vi "ck_clnt.vi"   [LabVIEW 2012]
uses:
  <vilib>/addons/internet/NI_InternetTK_Common_VIs.lvlib
  <vilib>/addons/internet/NI_InternetTK_Core_VIs.lvlib
types:
  T1 = typedef "CGI Connection Info.ctl" = cluster{"name":string, "type":T2, "session":T3}
  T2 = typedef "CGI Request Type.ctl" = enum16{"cgi", ".spool first", ".spool", ".spool last"}
  T3 = typedef "HTTP Session.ctl" = refnum<k1>
  T4 = typedef "NI_FTP.lvlib/Keyed Array.ctl" = cluster{"keys":string[], "values":string[]}
  T5 = typedef "Cookie.ctl" = cluster{"cookie id":string, "address":string}
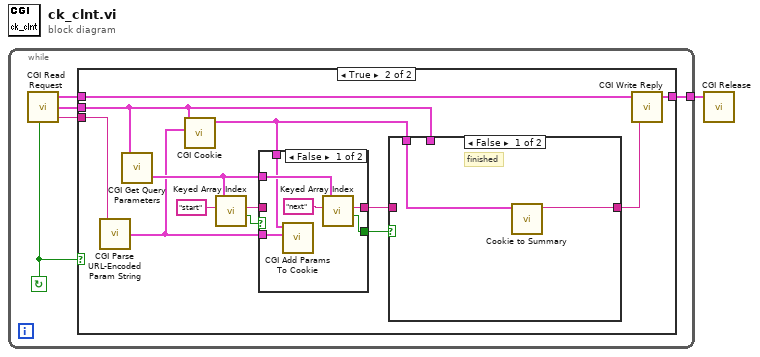
[diagram p0: block diagram]
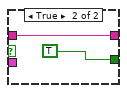
[diagram p3: hidden frame]
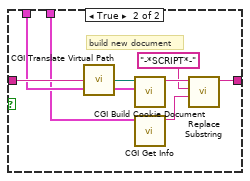
[diagram p4: hidden frame]
diagram:
  n1 = while {
    tunnel: [w2] -> w1
    stop <- w3 continue-if-true
    n2 = call <vilib>:"CGI Read Request.vi"() -> ("valid request?"=w3:bool, "cgi connection info"=w4:T1, "env"=w5:T4, "content"=w6:string)  [unwired: 4 in]
    n3 = case shown="True" w3 {
      tunnel: w4 -> [w7 w14]
      tunnel: [w7 w13] -> w2
      tunnel: w5 -> [_ w9]
      tunnel: w6 -> [_ w12]
      frame False {
      }
      frame True {
        n4 = call <vilib>:"CGI Parse URL-Encoded Param String.vi"("url-encoded param string"=w12) -> ("params"=w10:T4)
        n5 = call <vilib>:"CGI Get Query Parameters.vi"("env"=w9) -> ("query params"=w11:T4)  [unwired: 2 out]
        n6 = call <vilib>:"CGI Cookie.vi"("params"=w10, "env"=w9) -> ("cookie"=w8:T5)  [unwired: 6 in, 3 out]
        n7 = call <vilib>:"Keyed Array Index.vi"("key"="start", "array in"=w11) -> ("valid key"=w17:bool, "value"=w18:string)  [unwired: 3 in, 1 out]
        n8 = case shown="False" w17 {
          tunnel: w18 -> [_ w28]
          tunnel: w11 -> [w25 _]
          tunnel: [w24 TRUE ("valid key")] -> w19
          tunnel: [w23 w28] -> w20
          tunnel: w10 -> [w21 _]
          tunnel: w8 -> [w22 _]
          frame False {
            n9 = call <vilib>:"CGI Add Params To Cookie.vi"("params"=w21, "cookie"=w22) -> ()  [unwired: 8 in, 2 out]
            n10 = call <vilib>:"Keyed Array Index.vi"("key"="next", "array in"=w25) -> ("valid key"=w24:bool, "value"=w23:string)  [unwired: 3 in, 1 out]
          }
          frame True {
          }
        }
        n11 = case shown="False" w19 {
          tunnel: w20 -> [_ w38]
          tunnel: [w30 w35] -> w15
          tunnel: w9 -> [_ w32]
          tunnel: w8 -> [w29 w33]
          frame False {
            # "finished"
            n12 = call "Cookie to Summary.vi"("cookie"=w29) -> ("html summary"=w30:string)  [unwired: 9 in, 1 out]
          }
          frame True {
            # "build new document"
            n13 = call <vilib>:"CGI Translate Virtual Path.vi"("virtual path"=w38) -> ("absolute path"=w37:path)  [unwired: 1 in]
            n14 = call <vilib>:"CGI Build Cookie Document.vi"("cookie"=w33, "document path"=w37) -> ("parsed document"=w36:string)  [unwired: 7 in, 2 out]
            n15 = call <vilib>:"CGI Get Info.vi"("env"=w32) -> ("cgi name"=w31:string)  [unwired: 4 in, 2 out]
            n16 = call <vilib>:"Replace Substring.vi"("replacement"=w31, "pattern"="-*SCRIPT*-", "text"=w36) -> ("text out"=w35:string)  [unwired: 7 in, 1 out]
          }
        }
        n17 = call <vilib>:"CGI Write Reply.vi"("content"=w15, "cgi connection info"=w14) -> ("cgi connection info out"=w13:T1)  [unwired: 3 in]
      }
    }
  }
  n18 = call <vilib>:"CGI Release.vi"("cgi connection info"=w1) -> ()  [unwired: 5 in]
